vi "Merge two co-incident cells.vi"(10 "Grain 2":T1={"Structure Name"="Batch6_1", "Lattice vector a"=[9.1641, 0.0, 0.0], "Lattice vector b"=[0.0, 7.93635, 0.0], "Lattice vector c"=[0.0, 0.0, 17.5617], "Atoms Array"=[{"Atom Name"="Cd", "Positions (Direct)"=[[1e-06, 0.133333, 0.072927], [0.500001, 0.133333, 0.072927], [0.250001, 0.633333, 0.072927], [0.750001, 0.633333, 0.072927], [0.250001, 0.3, 0.285961], [0.750001, 0.3, 0.285961], [1e-06, 0.8, 0.285961], [0.500001, 0.8, 0.285961], [1e-06, 0.466667, 0.498995], [0.500001, 0.466667, 0.498995], [0.250001, 0.966667, 0.498995], [0.750001, 0.966667, 0.498995], [0.25, 0.134593, 0.662792], [0.75, 0.134593, 0.662792], [0.0, 0.634593, 0.662792], [0.5, 0.634593, 0.662792], [0.125, 0.467068, 0.873815], [0.625, 0.467068, 0.873815], [0.375, 0.967067, 0.873815], [0.875, 0.967067, 0.873815]], "Positions (Cartesian)"=[[9.1641e-06, 1.05817735455, 1.2807220959], [4.5820591641, 1.05817735455, 1.2807220959], [2.2910341640999996, 5.02635235455, 1.2807220959], [6.8730841641, 5.02635235455, 1.2807220959], [2.2910341640999996, 2.380905, 5.0219612936999996], [6.8730841641, 2.380905, 5.0219612936999996], [9.1641e-06, 6.349080000000001, 5.0219612936999996], [4.5820591641, 6.349080000000001, 5.0219612936999996], [9.1641e-06, 3.70363264545, 8.7632004915], [4.5820591641, 3.70363264545, 8.7632004915], [2.2910341640999996, 7.67180764545, 8.7632004915], [6.8730841641, 7.67180764545, 8.7632004915], [2.291025, 1.06817715555, 11.639754266399999], [6.873075, 1.06817715555, 11.639754266399999], [0.0, 5.0363521555499995, 11.639754266399999], [4.58205, 5.0363521555499995, 11.639754266399999], [1.1455125, 3.7068151218, 15.345676885499998], [5.7275624999999994, 3.7068151218, 15.345676885499998], [3.4365375, 7.67498218545, 15.345676885499998], [8.018587499999999, 7.67498218545, 15.345676885499998]]}, {"Atom Name"="Te", "Positions (Direct)"=[[0.250001, 0.3, 0.126185], [0.750001, 0.3, 0.126185], [1e-06, 0.8, 0.126185], [0.500001, 0.8, 0.126185], [1e-06, 0.466667, 0.339219], [0.500001, 0.466667, 0.339219], [0.250001, 0.966667, 0.339219], [0.750001, 0.966667, 0.339219], [1e-06, 0.133333, 0.552254], [0.500001, 0.133333, 0.552254], [0.250001, 0.633333, 0.552254], [0.750001, 0.633333, 0.552254], [0.25, 0.467926, 0.71605], [0.75, 0.467926, 0.71605], [0.0, 0.967926, 0.71605], [0.5, 0.967926, 0.71605], [0.125, 0.133735, 0.927073], [0.625, 0.133735, 0.927073], [0.375, 0.633734, 0.927073], [0.875, 0.633734, 0.927073]], "Positions (Cartesian)"=[[2.2910341640999996, 2.380905, 2.2160231144999996], [6.8730841641, 2.380905, 2.2160231144999996], [9.1641e-06, 6.349080000000001, 2.2160231144999996], [4.5820591641, 6.349080000000001, 2.2160231144999996], [9.1641e-06, 3.70363264545, 5.957262312299999], [4.5820591641, 3.70363264545, 5.957262312299999], [2.2910341640999996, 7.67180764545, 5.957262312299999], [6.8730841641, 7.67180764545, 5.957262312299999], [9.1641e-06, 1.05817735455, 9.6985190718], [4.5820591641, 1.05817735455, 9.6985190718], [2.2910341640999996, 5.02635235455, 9.6985190718], [6.8730841641, 5.02635235455, 9.6985190718], [2.291025, 3.7136245101000003, 12.575055284999998], [6.873075, 3.7136245101000003, 12.575055284999998], [0.0, 7.681799510099999, 12.575055284999998], [4.58205, 7.681799510099999, 12.575055284999998], [1.1455125, 1.06136776725, 16.2809779041], [5.7275624999999994, 1.06136776725, 16.2809779041], [3.4365375, 5.0295348309, 16.2809779041], [8.018587499999999, 5.0295348309, 16.2809779041]]}], "# of atoms"=40}, 11 "Grain 1":T1={"Structure Name"="Batch6_1", "Lattice vector a"=[9.1641, 0.0, 0.0], "Lattice vector b"=[0.0, 7.93635, 0.0], "Lattice vector c"=[0.0, 0.0, 17.5617], "Atoms Array"=[{"Atom Name"="Cd", "Positions (Direct)"=[[1e-06, 0.133333, 0.072927], [0.500001, 0.133333, 0.072927], [0.250001, 0.633333, 0.072927], [0.750001, 0.633333, 0.072927], [0.250001, 0.3, 0.285961], [0.750001, 0.3, 0.285961], [1e-06, 0.8, 0.285961], [0.500001, 0.8, 0.285961], [1e-06, 0.466667, 0.498995], [0.500001, 0.466667, 0.498995], [0.250001, 0.966667, 0.498995], [0.750001, 0.966667, 0.498995], [0.25, 0.134593, 0.662792], [0.75, 0.134593, 0.662792], [0.0, 0.634593, 0.662792], [0.5, 0.634593, 0.662792], [0.125, 0.467068, 0.873815], [0.625, 0.467068, 0.873815], [0.375, 0.967067, 0.873815], [0.875, 0.967067, 0.873815]], "Positions (Cartesian)"=[[9.1641e-06, 1.05817735455, 1.2807220959], [4.5820591641, 1.05817735455, 1.2807220959], [2.2910341640999996, 5.02635235455, 1.2807220959], [6.8730841641, 5.02635235455, 1.2807220959], [2.2910341640999996, 2.380905, 5.0219612936999996], [6.8730841641, 2.380905, 5.0219612936999996], [9.1641e-06, 6.349080000000001, 5.0219612936999996], [4.5820591641, 6.349080000000001, 5.0219612936999996], [9.1641e-06, 3.70363264545, 8.7632004915], [4.5820591641, 3.70363264545, 8.7632004915], [2.2910341640999996, 7.67180764545, 8.7632004915], [6.8730841641, 7.67180764545, 8.7632004915], [2.291025, 1.06817715555, 11.639754266399999], [6.873075, 1.06817715555, 11.639754266399999], [0.0, 5.0363521555499995, 11.639754266399999], [4.58205, 5.0363521555499995, 11.639754266399999], [1.1455125, 3.7068151218, 15.345676885499998], [5.7275624999999994, 3.7068151218, 15.345676885499998], [3.4365375, 7.67498218545, 15.345676885499998], [8.018587499999999, 7.67498218545, 15.345676885499998]]}, {"Atom Name"="Te", "Positions (Direct)"=[[0.250001, 0.3, 0.126185], [0.750001, 0.3, 0.126185], [1e-06, 0.8, 0.126185], [0.500001, 0.8, 0.126185], [1e-06, 0.466667, 0.339219], [0.500001, 0.466667, 0.339219], [0.250001, 0.966667, 0.339219], [0.750001, 0.966667, 0.339219], [1e-06, 0.133333, 0.552254], [0.500001, 0.133333, 0.552254], [0.250001, 0.633333, 0.552254], [0.750001, 0.633333, 0.552254], [0.25, 0.467926, 0.71605], [0.75, 0.467926, 0.71605], [0.0, 0.967926, 0.71605], [0.5, 0.967926, 0.71605], [0.125, 0.133735, 0.927073], [0.625, 0.133735, 0.927073], [0.375, 0.633734, 0.927073], [0.875, 0.633734, 0.927073]], "Positions (Cartesian)"=[[2.2910341640999996, 2.380905, 2.2160231144999996], [6.8730841641, 2.380905, 2.2160231144999996], [9.1641e-06, 6.349080000000001, 2.2160231144999996], [4.5820591641, 6.349080000000001, 2.2160231144999996], [9.1641e-06, 3.70363264545, 5.957262312299999], [4.5820591641, 3.70363264545, 5.957262312299999], [2.2910341640999996, 7.67180764545, 5.957262312299999], [6.8730841641, 7.67180764545, 5.957262312299999], [9.1641e-06, 1.05817735455, 9.6985190718], [4.5820591641, 1.05817735455, 9.6985190718], [2.2910341640999996, 5.02635235455, 9.6985190718], [6.8730841641, 5.02635235455, 9.6985190718], [2.291025, 3.7136245101000003, 12.575055284999998], [6.873075, 3.7136245101000003, 12.575055284999998], [0.0, 7.681799510099999, 12.575055284999998], [4.58205, 7.681799510099999, 12.575055284999998], [1.1455125, 1.06136776725, 16.2809779041], [5.7275624999999994, 1.06136776725, 16.2809779041], [3.4365375, 5.0295348309, 16.2809779041], [8.018587499999999, 5.0295348309, 16.2809779041]]}], "# of atoms"=40}) -> (3 "Joined GB":T1={"Structure Name"="Batch6_1+Batch6_1", "Lattice vector a"=[9.1641, 0.0, 0.0], "Lattice vector b"=[0.0, 7.93635, 0.0], "Lattice vector c"=[0.0, 0.0, 35.1234], "Atoms Array"=[{"Atom Name"="Cd", "Positions (Direct)"=[[1e-06, 0.13333299999999998, 0.03646350000000001], [0.500001, 0.13333299999999998, 0.03646350000000001], [0.250001, 0.6333329999999999, 0.03646350000000001], [0.750001, 0.6333329999999999, 0.03646350000000001], [0.250001, 0.29999999999999993, 0.1429805], [0.750001, 0.29999999999999993, 0.1429805], [1e-06, 0.8, 0.1429805], [0.500001, 0.8, 0.1429805], [1e-06, 0.46666699999999994, 0.2494975], [0.500001, 0.46666699999999994, 0.2494975], [0.250001, 0.9666669999999999, 0.2494975], [0.750001, 0.9666669999999999, 0.2494975], [0.25, 0.134593, 0.331396], [0.75, 0.134593, 0.331396], [0.0, 0.6345929999999999, 0.331396], [0.5, 0.6345929999999999, 0.331396], [0.125, 0.467068, 0.4369075], [0.625, 0.467068, 0.4369075], [0.375, 0.9670669999999999, 0.4369075], [0.8749999999999999, 0.9670669999999999, 0.4369075], [1e-06, 0.13333299999999998, 0.5364635], [0.500001, 0.13333299999999998, 0.5364635], [0.250001, 0.6333329999999999, 0.5364635], [0.750001, 0.6333329999999999, 0.5364635], [0.250001, 0.29999999999999993, 0.6429805], [0.750001, 0.29999999999999993, 0.6429805], [1e-06, 0.8, 0.6429805], [0.500001, 0.8, 0.6429805], [1e-06, 0.46666699999999994, 0.7494974999999999], [0.500001, 0.46666699999999994, 0.7494974999999999], [0.250001, 0.9666669999999999, 0.7494974999999999], [0.750001, 0.9666669999999999, 0.7494974999999999], [0.25, 0.134593, 0.831396], [0.75, 0.134593, 0.831396], [0.0, 0.6345929999999999, 0.831396], [0.5, 0.6345929999999999, 0.831396], [0.125, 0.467068, 0.9369075000000001], [0.625, 0.467068, 0.9369075000000001], [0.375, 0.9670669999999999, 0.9369075000000001], [0.8749999999999999, 0.9670669999999999, 0.9369075000000001]], "Positions (Cartesian)"=[[9.1641e-06, 1.05817735455, 1.2807220959], [4.5820591641, 1.05817735455, 1.2807220959], [2.2910341640999996, 5.02635235455, 1.2807220959], [6.8730841641, 5.02635235455, 1.2807220959], [2.2910341640999996, 2.380905, 5.0219612936999996], [6.8730841641, 2.380905, 5.0219612936999996], [9.1641e-06, 6.349080000000001, 5.0219612936999996], [4.5820591641, 6.349080000000001, 5.0219612936999996], [9.1641e-06, 3.70363264545, 8.7632004915], [4.5820591641, 3.70363264545, 8.7632004915], [2.2910341640999996, 7.67180764545, 8.7632004915], [6.8730841641, 7.67180764545, 8.7632004915], [2.291025, 1.06817715555, 11.639754266399999], [6.873075, 1.06817715555, 11.639754266399999], [0.0, 5.0363521555499995, 11.639754266399999], [4.58205, 5.0363521555499995, 11.639754266399999], [1.1455125, 3.7068151218, 15.345676885499998], [5.7275624999999994, 3.7068151218, 15.345676885499998], [3.4365375, 7.67498218545, 15.345676885499998], [8.018587499999999, 7.67498218545, 15.345676885499998], [9.1641e-06, 1.05817735455, 18.842422095899998], [4.5820591641, 1.05817735455, 18.842422095899998], [2.2910341640999996, 5.02635235455, 18.842422095899998], [6.8730841641, 5.02635235455, 18.842422095899998], [2.2910341640999996, 2.380905, 22.583661293699997], [6.8730841641, 2.380905, 22.583661293699997], [9.1641e-06, 6.349080000000001, 22.583661293699997], [4.5820591641, 6.349080000000001, 22.583661293699997], [9.1641e-06, 3.70363264545, 26.324900491499996], [4.5820591641, 3.70363264545, 26.324900491499996], [2.2910341640999996, 7.67180764545, 26.324900491499996], [6.8730841641, 7.67180764545, 26.324900491499996], [2.291025, 1.06817715555, 29.2014542664], [6.873075, 1.06817715555, 29.2014542664], [0.0, 5.0363521555499995, 29.2014542664], [4.58205, 5.0363521555499995, 29.2014542664], [1.1455125, 3.7068151218, 32.9073768855], [5.7275624999999994, 3.7068151218, 32.9073768855], [3.4365375, 7.67498218545, 32.9073768855], [8.018587499999999, 7.67498218545, 32.9073768855]]}, {"Atom Name"="Te", "Positions (Direct)"=[[0.250001, 0.29999999999999993, 0.0630925], [0.750001, 0.29999999999999993, 0.0630925], [1e-06, 0.8, 0.0630925], [0.500001, 0.8, 0.0630925], [1e-06, 0.46666699999999994, 0.1696095], [0.500001, 0.46666699999999994, 0.1696095], [0.250001, 0.9666669999999999, 0.1696095], [0.750001, 0.9666669999999999, 0.1696095], [1e-06, 0.13333299999999998, 0.276127], [0.500001, 0.13333299999999998, 0.276127], [0.250001, 0.6333329999999999, 0.276127], [0.750001, 0.6333329999999999, 0.276127], [0.25, 0.467926, 0.358025], [0.75, 0.467926, 0.358025], [0.0, 0.9679259999999998, 0.358025], [0.5, 0.9679259999999998, 0.358025], [0.125, 0.133735, 0.4635365], [0.625, 0.133735, 0.4635365], [0.375, 0.633734, 0.4635365], [0.8749999999999999, 0.633734, 0.4635365], [0.250001, 0.29999999999999993, 0.5630925], [0.750001, 0.29999999999999993, 0.5630925], [1e-06, 0.8, 0.5630925], [0.500001, 0.8, 0.5630925], [1e-06, 0.46666699999999994, 0.6696095], [0.500001, 0.46666699999999994, 0.6696095], [0.250001, 0.9666669999999999, 0.6696095], [0.750001, 0.9666669999999999, 0.6696095], [1e-06, 0.13333299999999998, 0.776127], [0.500001, 0.13333299999999998, 0.776127], [0.250001, 0.6333329999999999, 0.776127], [0.750001, 0.6333329999999999, 0.776127], [0.25, 0.467926, 0.858025], [0.75, 0.467926, 0.858025], [0.0, 0.9679259999999998, 0.858025], [0.5, 0.9679259999999998, 0.858025], [0.125, 0.133735, 0.9635365000000001], [0.625, 0.133735, 0.9635365000000001], [0.375, 0.633734, 0.9635365000000001], [0.8749999999999999, 0.633734, 0.9635365000000001]], "Positions (Cartesian)"=[[2.2910341640999996, 2.380905, 2.2160231144999996], [6.8730841641, 2.380905, 2.2160231144999996], [9.1641e-06, 6.349080000000001, 2.2160231144999996], [4.5820591641, 6.349080000000001, 2.2160231144999996], [9.1641e-06, 3.70363264545, 5.957262312299999], [4.5820591641, 3.70363264545, 5.957262312299999], [2.2910341640999996, 7.67180764545, 5.957262312299999], [6.8730841641, 7.67180764545, 5.957262312299999], [9.1641e-06, 1.05817735455, 9.6985190718], [4.5820591641, 1.05817735455, 9.6985190718], [2.2910341640999996, 5.02635235455, 9.6985190718], [6.8730841641, 5.02635235455, 9.6985190718], [2.291025, 3.7136245101000003, 12.575055284999998], [6.873075, 3.7136245101000003, 12.575055284999998], [0.0, 7.681799510099999, 12.575055284999998], [4.58205, 7.681799510099999, 12.575055284999998], [1.1455125, 1.06136776725, 16.2809779041], [5.7275624999999994, 1.06136776725, 16.2809779041], [3.4365375, 5.0295348309, 16.2809779041], [8.018587499999999, 5.0295348309, 16.2809779041], [2.2910341640999996, 2.380905, 19.7777231145], [6.8730841641, 2.380905, 19.7777231145], [9.1641e-06, 6.349080000000001, 19.7777231145], [4.5820591641, 6.349080000000001, 19.7777231145], [9.1641e-06, 3.70363264545, 23.518962312299998], [4.5820591641, 3.70363264545, 23.518962312299998], [2.2910341640999996, 7.67180764545, 23.518962312299998], [6.8730841641, 7.67180764545, 23.518962312299998], [9.1641e-06, 1.05817735455, 27.260219071799998], [4.5820591641, 1.05817735455, 27.260219071799998], [2.2910341640999996, 5.02635235455, 27.260219071799998], [6.8730841641, 5.02635235455, 27.260219071799998], [2.291025, 3.7136245101000003, 30.136755284999996], [6.873075, 3.7136245101000003, 30.136755284999996], [0.0, 7.681799510099999, 30.136755284999996], [4.58205, 7.681799510099999, 30.136755284999996], [1.1455125, 1.06136776725, 33.8426779041], [5.7275624999999994, 1.06136776725, 33.8426779041], [3.4365375, 5.0295348309, 33.8426779041], [8.018587499999999, 5.0295348309, 33.8426779041]]}], "# of atoms"=80})   [LabVIEW 2010]
panel:
  out "Array":i32[](array[numeric])
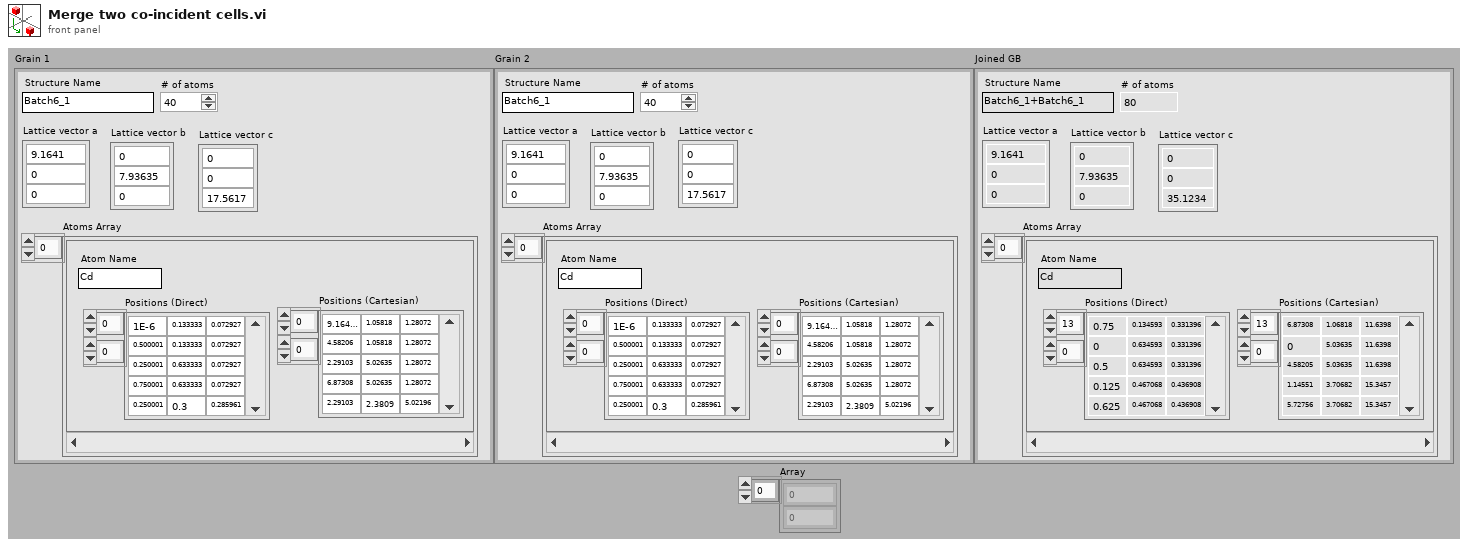
[diagram p1: front panel]
types:
  T1 = cluster{"Structure Name":string, "Lattice vector a":dbl[], "Lattice vector b":dbl[], "Lattice vector c":dbl[], "Atoms Array":cluster{"Atom Name":string, "Positions (Direct)":dbl[][], "Positions (Cartesian)":dbl[][]}[], "# of atoms":i32}
  T2 = cluster{"Atom Name":string, "Positions (Direct)":dbl[][], "Positions (Cartesian)":dbl[][]}[]
  T3 = cluster{"Structure Name":string, "Lattice vector a":dbl[], "Lattice vector b":dbl[], dbl[], cluster{"Atom Name":string, dbl[][], dbl[][]}[], i32}
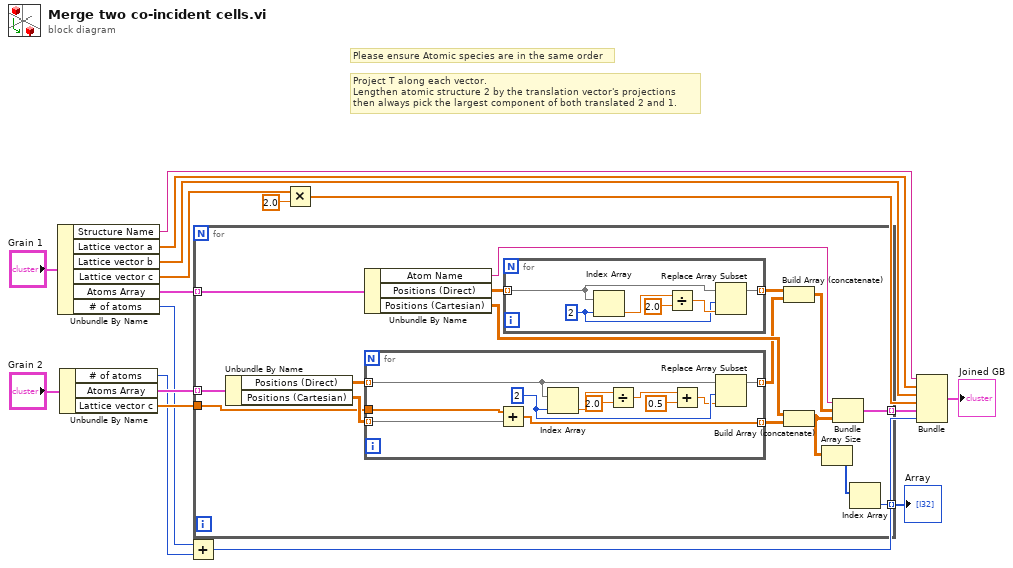
[diagram p0: block diagram]
diagram:
  # "Project T along each vector.\nLengthen atomic structure 2 by the translation vector's projections\nthen always pick the largest component of both translated 2 and 1."
  # "Please ensure Atomic species are in the same order"
  n1 = Unbundle By Name("Grain 1") -> ("Structure Name"=w9:string, "Lattice vector a"=w8:dbl[], "Lattice vector b"=w7:dbl[], "Lattice vector c"=w5:dbl[], "Atoms Array"=w13:T2, "# of atoms"=w10:i32)
  n2 = Unbundle By Name("Grain 2") -> ("# of atoms"=w11:i32, "Atoms Array"=w14:T2, "Lattice vector c"=w12:dbl[])
  n3 = Add(x=w10, y=w11) -> (x+y=w2:i32)
  n4 = for {
    tunnel: w14 -> [w32] mode=indexing
    tunnel: w13 -> [w33] mode=indexing
    tunnel: w12 -> [w29]
    tunnel: [w21] -> w3 mode=indexing
    tunnel: [w18] -> w1 mode=indexing
    n5 = Unbundle By Name(w32) -> ("Positions (Direct)"=w26:dbl[][], "Positions (Cartesian)"=w30:dbl[][])
    n6 = Unbundle By Name(w33) -> ("Atom Name"=w22:string, "Positions (Direct)"=w31:dbl[][], "Positions (Cartesian)"=w27:dbl[][])
    n7 = for {
      tunnel: w30 -> [w43] mode=indexing
      tunnel: w29 -> [w44]
      tunnel: [w42] -> w28 mode=indexing
      tunnel: w26 -> [w38] mode=indexing
      tunnel: [w34] -> w24 mode=indexing
      w39 = 2 ("index")
      n8 = Add(x=w44, y=w43) -> (x+y=w42:dbl[])
      n9 = Index Array(array=w38, index=w39) -> (element=w40:dbl)
      n10 = Divide(x=w40, y=2.0) -> (x/y=w37:dbl)
      n11 = Add(x=w37, y=0.5) -> (x+y=w35:dbl)
      n12 = Replace Array Subset(array=w38, new element=w35, index=w39) -> (w34:dbl[])
    }
    n13 = for {
      tunnel: w31 -> [w48] mode=indexing
      tunnel: [w45] -> w25 mode=indexing
      w46 = 2 ("index")
      n14 = Index Array(array=w48, index=w46) -> (element=w49:dbl)
      n15 = Divide(x=w49, y=2.0) -> (x/y=w47:dbl)
      n16 = Replace Array Subset(array=w48, new element=w47, index=w46) -> (w45:dbl[])
    }
    n17 = Build Array (concatenate)(w25, w24) -> (w23:dbl[][])
    n18 = Build Array (concatenate)(w27, w28) -> (w20:dbl[][])
    n19 = Array Size(array=w20) -> (size(s)=w19:i32[])
    n20 = Bundle("Atom Name"=w22, w23, w20) -> (w21:cluster{"Atom Name":string, dbl[][], dbl[][]})  [unwired: 1 in]
    n21 = Index Array(array=w19) -> (element=w18:i32)  [unwired: 1 in]
  }
  "Array" <- w1
  n22 = Multiply(x=w5, y=2.0) -> (x*y=w4:dbl[])
  n23 = Bundle("Structure Name"=w9, "Lattice vector a"=w8, "Lattice vector b"=w7, w4, w3, w2) -> (→"Joined GB":T3)  [unwired: 1 in]
